vi "Binomial PF.vi"(9 "p":dbl=0.02, 10 "n":i32=100, 11 "x":i32) -> (0 "error":i32, 3 "prob(x)":dbl=0.13261955589475294)   [LabVIEW 2020, in "NI_Gmath.lvlib"]
doc: "Computes the discrete probability function (PF), or the probability that the random variate X, where X describes the selected distribution type, takes on the value <B>n</B>. You must manually select the polymorphic instance to use."
uses:
  NI_Gmath.lvlib
panel:
  # "Binomial PF"
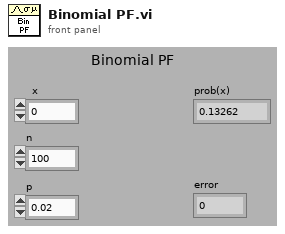
[diagram p1: front panel]
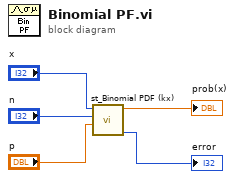
[diagram p0: block diagram]
diagram:
  n1 = call "st_Binomial PDF (kx).vi"("p"="p", "n"="n", "x"="x") -> ("error"=→"error":i32, "pdf(x)"=→"prob(x)":dbl)  [unwired: 7 in]
